vi "Count_independent.vi"(7 "Reset?":bool[](array[boolean]), 11 "Input array":dbl[](array[numeric])) -> (3 "Output array":dbl[](array[numeric]))   [LabVIEW 2018]
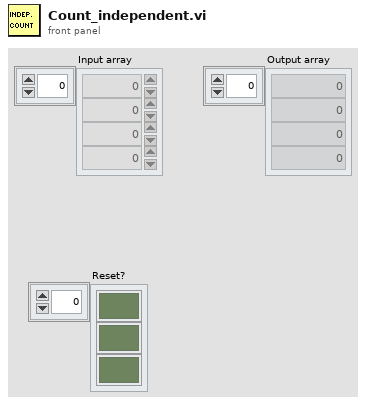
[diagram p1: front panel]
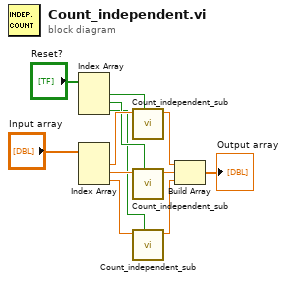
[diagram p0: block diagram]
diagram:
  n1 = Index Array(array="Reset?") -> (element #1=w3:bool, element #2=w2:bool, element #3=w1:bool)  [unwired: 3 in]
  n2 = Index Array(array="Input array") -> (element #1=w11:dbl, element #2=w10:dbl, element #3=w9:dbl)  [unwired: 3 in]
  n3 = call "Count_independent_sub.vi"("Reset?"=w3, "Input sample"=w11) -> ("Sum of samples"=w8:dbl)  [unwired: 9 in]
  n4 = call "Count_independent_sub.vi"("Reset?"=w2, "Input sample"=w10) -> ("Sum of samples"=w7:dbl)  [unwired: 9 in]
  n5 = call "Count_independent_sub.vi"("Reset?"=w1, "Input sample"=w9) -> ("Sum of samples"=w6:dbl)  [unwired: 9 in]
  n6 = Build Array(w8, w7, w6) -> (→"Output array":dbl[])
